vi "ManageLEDs.vi"(9 "Right thickness in range?":bool, 10 "Left thickness in range?":bool, 11 "Average thickness in range?":bool) -> ()   [LabVIEW 2013]
uses:
  Global.vi
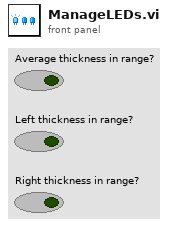
[diagram p1: front panel]
types:
  T1 = cluster{"Good average":refnum<vi>, "Good right":refnum<vi>, "Good left":refnum<vi>, "Bad average":refnum<vi>, "Bad right":refnum<vi>, "Bad left":refnum<vi>}
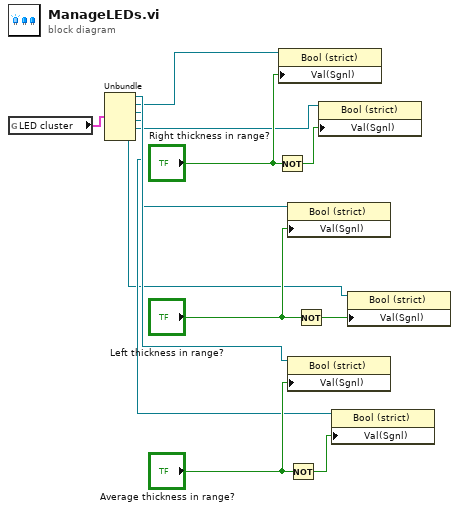
[diagram p0: block diagram]
diagram:
  n1 = global read "Global.vi" "LED cluster"() -> (w7:T1)
  n2 = Unbundle(w7) -> ("Good average"=w6:refnum<vi>, "Good right"=w5:refnum<vi>, "Good left"=w4:refnum<vi>, "Bad average"=w3:refnum<vi>, "Bad right"=w2:refnum<vi>, "Bad left"=w1:refnum<vi>)
  n3 = Not(x="Right thickness in range?") -> (.not. x?=w12:bool)
  n4 = property class="Bool (strict)"(reference=w5, "Val(Sgnl)"="Right thickness in range?") -> ()  [unwired: 1 in, 2 out]
  n5 = property class="Bool (strict)"(reference=w4, "Val(Sgnl)"="Left thickness in range?") -> ()  [unwired: 1 in, 2 out]
  n6 = property class="Bool (strict)"(reference=w6, "Val(Sgnl)"="Average thickness in range?") -> ()  [unwired: 1 in, 2 out]
  n7 = Not(x="Average thickness in range?") -> (.not. x?=w8:bool)
  n8 = Not(x="Left thickness in range?") -> (.not. x?=w9:bool)
  n9 = property class="Bool (strict)"(reference=w2, "Val(Sgnl)"=w12) -> ()  [unwired: 1 in, 2 out]
  n10 = property class="Bool (strict)"(reference=w3, "Val(Sgnl)"=w8) -> ()  [unwired: 1 in, 2 out]
  n11 = property class="Bool (strict)"(reference=w1, "Val(Sgnl)"=w9) -> ()  [unwired: 1 in, 2 out]
